vi "DAQ_StopTask.vi"(8 "error in (no error)":errorcluster, 10 "Message Enqueuer":refnum<class "Message Enqueuer.lvclass">, 11 "Task":string) -> (0 "error out":errorcluster)   [LabVIEW 2025, in "DAQ_API.lvlib"]
uses:
  DAQ_API.lvlib
  <vilib>/ActorFramework/Message Enqueuer/Message Enqueuer.lvclass
  DAQ_Module/DAQ_Module/DAQ_Module Messages/StopTask Msg/StopTask Msg.lvclass/StopTask Msg.ctl
  <vilib>/ActorFramework/Message Enqueuer/Message Enqueuer.lvclass/Message Enqueuer.ctl
  <vilib>/ActorFramework/Message Enqueuer/Enqueue.vi
  DAQ_Module/DAQ_Module/DAQ_Module Messages/StopTask Msg/StopTask Msg.lvclass
  C:/Program Files (x86)/National Instruments/LabVIEW 2025/vi.lib/ActorFramework/Message/Message.lvclass
  <vilib>/ActorFramework/Message Priority Queue/Priority Enqueue.vi
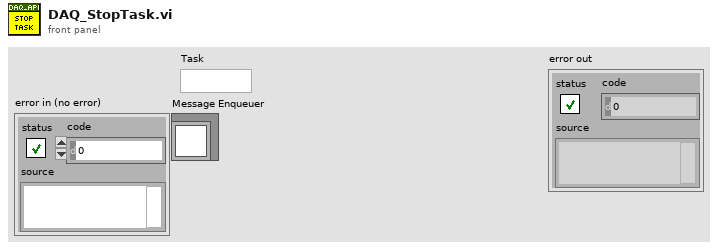
[diagram p1: front panel]
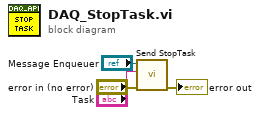
[diagram p0: block diagram]
diagram:
  n1 = call "Send StopTask.vi"("error in (no error)"="error in (no error)", "Task"="Task", "Message Enqueuer"="Message Enqueuer") -> ("error out"=→"error out":errorcluster)  [unwired: 7 in, 1 out]
